vi "Save_current_setup.vi"(3 "Save New File?":bool, 5 "Setup File Type":T1) -> (0 "Cancelled?":bool, 1 "Saved filepath":path, 2 "Current Setup":path)   [LabVIEW 2015]
uses:
  File/Setup_Filetype.ctl
  Data_plotting_vis/Results_plotter_Global.vi
panel:
  out "Existing Setup names":string[](array[string])
  in  "New Setup filename":string
  in  "Cancel Button":bool
  in  "OK":bool
  # "To re-use an existing filename, copy and paste from the array at the left"
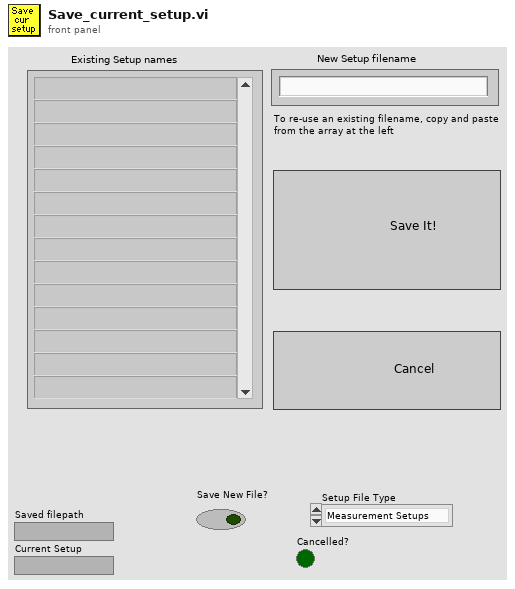
[diagram p1: front panel]
types:
  T1 = typedef "Setup_Filetype.ctl" = enum16{"Measurement Setups", "Calibration Setups", "General", "Results File Plotter Setups", "Speed Calib Tweaks"}
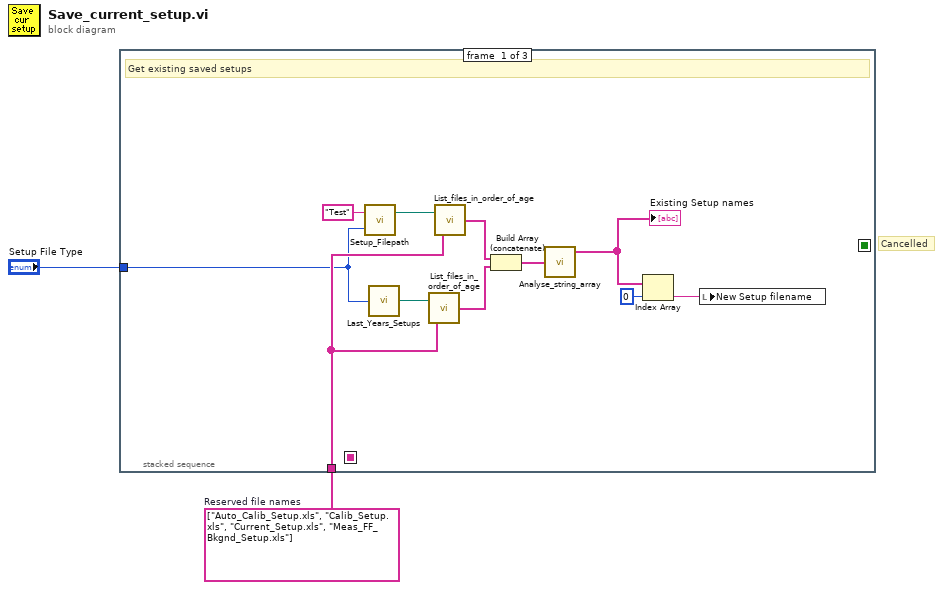
[diagram p0: block diagram]
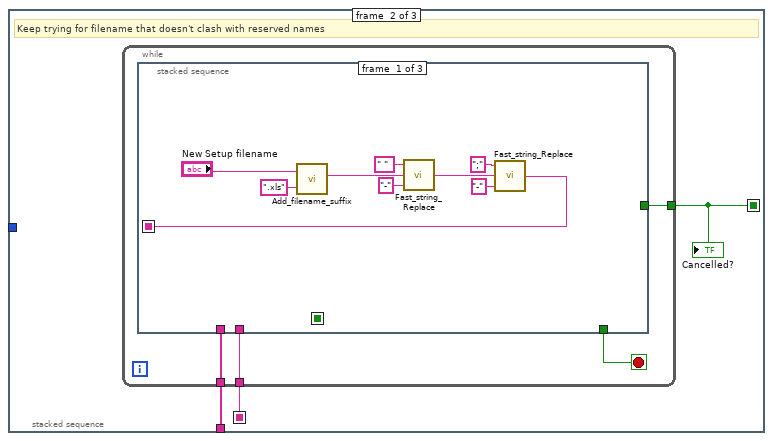
[diagram p2: hidden frame]
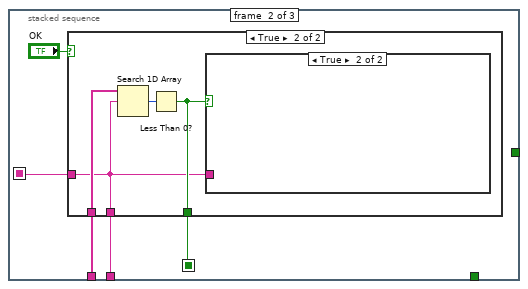
[diagram p3: hidden frame]
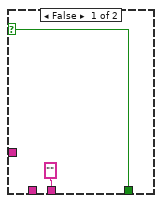
[diagram p4: hidden frame]
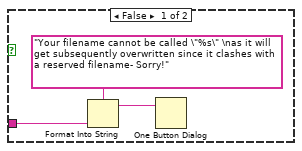
[diagram p5: hidden frame]
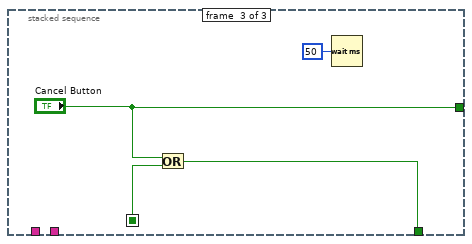
[diagram p6: hidden frame]
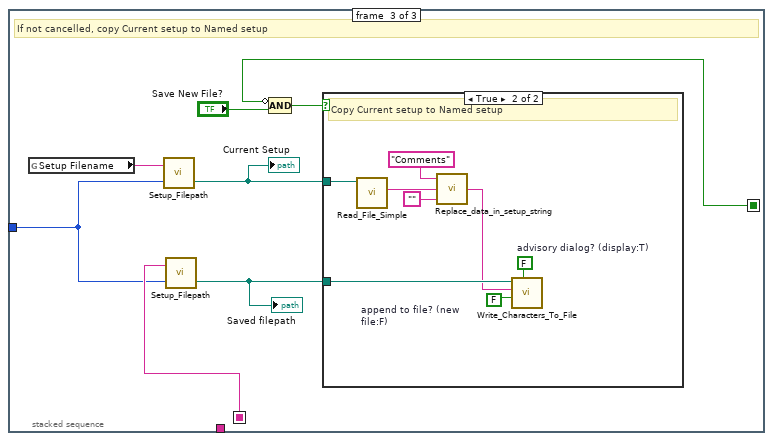
[diagram p7: hidden frame]
diagram:
  w2 = string[] ["Auto_Calib_Setup.xls", "Calib_Setup.xls", "Current_Setup.xls", "Meas_FF_Bkgnd_Setup.xls"]  # Reserved file names
  # "Cancelled"
  n1 = stacked-sequence {
    seq-local: [_ w16 _] -> [_ _ w51]
    seq-local: [_ w15 _] -> [_ _ w55]
    tunnel: w2 -> [w11 w14 _]
    tunnel: "Setup File Type" -> [w5 _ w49]
    frame #0 {
      # "Get existing saved setups"
      n2 = call "Setup_Filepath.vi"("Setup File Type"=w5, "Filename in"="Test") -> ("Directory"=w9:path)  [unwired: 1 out]
      n3 = call "Last_Years_Setups.vi"("Setup File Type"=w5) -> ("Directory"=w10:path)
      n4 = call "List_files_in_order_of_age.vi"("Files to Hide"=w11, "Folder"=w10) -> ("file names"=w7:string[])
      n5 = call "List_files_in_order_of_age.vi"("Files to Hide"=w11, "Folder"=w9) -> ("file names"=w8:string[])
      n6 = Build Array (concatenate)(w8, w7) -> (w4:string[])
      n7 = call "Analyse_string_array.vi"("String array"=w4) -> ("Unique strings"=w3:string[])  [unwired: 1 in, 1 out]
      "Existing Setup names" <- w3
      n8 = Index Array(array=w3, index=0) -> (element=w12:string)
      n9 = local write "New Setup filename"(w12) -> ()
    }
    frame #1 {
      # "Keep trying for filename that doesn't clash with reserved names"
      n10 = while {
        tunnel: [w20] -> w16
        tunnel: [w18] -> w15
        tunnel: w14 -> [w17]
        stop <- w19 stop-if-true
        n11 = stacked-sequence {
          seq-local: [w22 _ _] -> [_ w34 _]
          seq-local: [_ w32 _] -> [_ _ w47]
          tunnel: [_ w33 _] -> w20
          tunnel: [_ _ w46] -> w19
          tunnel: [_ _ "Cancel Button"] -> w18
          tunnel: w17 -> [_ w30 _]
          frame #0 {
            n12 = call "Add_filename_suffix.vi"("Filename"="New Setup filename", "Suffix to add"=".xls") -> ("Filename out"=w27:string)  [unwired: 3 out]
            n13 = call "Fast_string_Replace.vi"("Replace match with:"="-", "Input String"=w27, "regular expression"=" ") -> ("Output String"=w23:string)  [unwired: 2 out]
            n14 = call "Fast_string_Replace.vi"("Replace match with:"="-", "Input String"=w23, "regular expression"=";") -> ("Output String"=w22:string)  [unwired: 2 out]
          }
          frame #1 {
            n15 = case shown="True" "OK" {
              selector: "OK" -> [w35 _]
              tunnel: w34 -> [_ w37]
              tunnel: [w35 w38] -> w32
              tunnel: ["" ("File name only") w37] -> w33
              tunnel: w30 -> [_ w40]
              frame False {
              }
              frame True {
                n16 = Search 1D Array(1D array=w40, element=w37) -> (index of element=w39:i32)  [unwired: 1 out]
                n17 = Less Than 0?(x=w39) -> (x < 0?=w38:bool)
                n18 = case shown="True" w38 {
                  tunnel: w37 -> [w42 _]
                  frame False {
                    n19 = Format Into String(format string="Your filename cannot be called \"%s\" \nas it will get subsequently overwritten since it clashes with a reserved filename- Sorry!", w42) -> (resulting string=w41:string)  [unwired: 2 in, 1 out]
                    n20 = One Button Dialog(message=w41) -> ()  [unwired: 2 out]
                  }
                  frame True {
                  }
                }
              }
            }
          }
          frame #2 {
            n21 = Or(x="Cancel Button", y=w47) -> (x .or. y?=w46:bool)
            n22 = Wait (ms)(milliseconds to wait=u32 50) -> ()  [unwired: 1 out]
          }
        }
      }
      "Cancelled?" <- w15
    }
    frame #2 {
      # "If not cancelled, copy Current setup to Named setup"
      n23 = global read "Results_plotter_Global.vi" "Setup Filename"() -> (w48:string)
      n24 = call "Setup_Filepath.vi"("Setup File Type"=w49, "Filename in"=w48) -> ("Filename Out"=w52:path)  [unwired: 1 out]
      "Current Setup" <- w52
      n25 = call "Setup_Filepath.vi"("Setup File Type"=w49, "Filename in"=w51) -> ("Filename Out"=w50:path)  [unwired: 1 out]
      "Saved filepath" <- w50
      n26 = Compound Arithmetic op=AND(invert w55, "Save New File?") -> (w53:bool)
      n27 = case shown="True" w53 {
        tunnel: w52 -> [_ w63]
        tunnel: w50 -> [_ w62]
        frame False {
        }
        frame True {
          w60 = FALSE  # advisory dialog? (display:T)
          w61 = FALSE  # append to file? (new file:F)
          # "Copy Current setup to Named setup"
          n28 = call "Read_File_Simple.vi"("Filename"=w63) -> ("string"=w57:string)  [unwired: 2 in, 7 out]
          n29 = call "Replace_data_in_setup_string.vi"("New data string"="", "Input string"=w57, "Variable name"="Comments") -> ("Appended string"=w56:string)
          n30 = call "Write_Characters_To_File.vi"("file path (dialog if empty)"=w62, "advisory dialog? (display:T)"=w60, "character string"=w56, "append to file? (new file:F)"=w61) -> ()  [unwired: 1 in, 4 out]
        }
      }
    }
  }
